vi "run.vi"(8 "error in (no error)":errorcluster, 11 "GenericDisplay in":refnum<class "GenericDisplay.lvclass">) -> (0 "error out":errorcluster, 3 "GenericDisplay out":refnum<class "GenericDisplay.lvclass">)   [LabVIEW 2010, in "GenericDisplay.lvclass"]
uses:
  GenericDisplay.lvclass
panel:
  # "Functionality not available..."
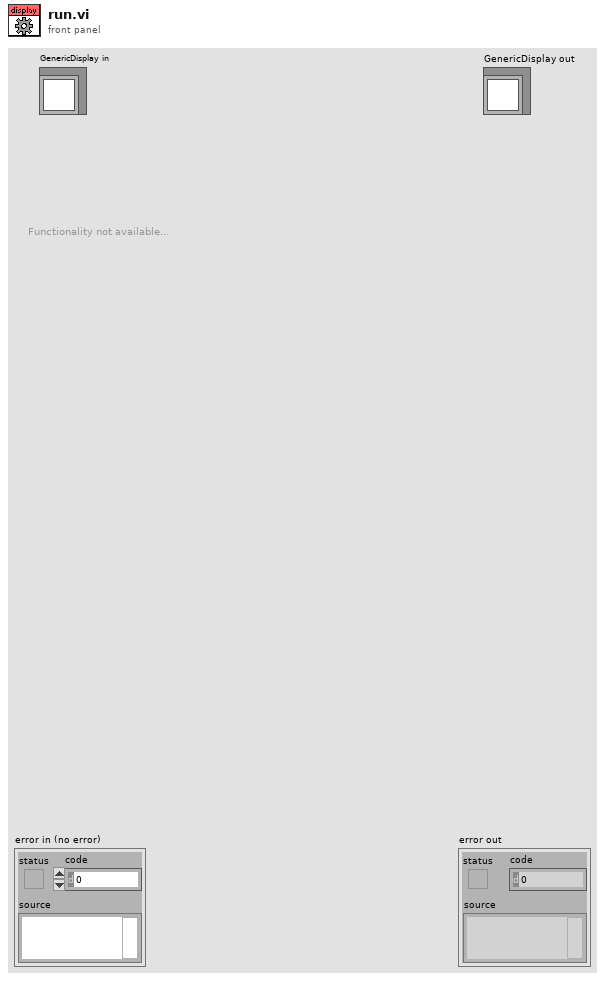
[diagram p1: front panel]
types:
  T1 = typedef "main_trigger_enum.ctl" = enum16{"NULL", "initialise", "terminate", "start", "stop", "change objective", "change experimentController", "change imagingMode", "save notebook", "started saving", "finished saving", "expCtr ready", "expCtr missing", "imgMd ready", "imgMd missing", "scanHd ready", "scanHd missing", "DAQ ready", "DAQ missing", "imgAsm ready", "imgAsm missing", "dataColl ready", "dataColl missing", "display ready", "display missing", "analysr ready", "analysr missing", "instrmnt ready", "instrmnt missing", "stimltr ready", "stimltr missing", "stage ready", "stage missing"}
  T2 = typedef "GenericToplevelComponent.lvclass/common_trigger_enum.ctl" = enum16{"NULL", "initialise", "terminate", "fetch command", "fetch data", "attach observer", "register as observer", "detach observer", "acknowledge", "start", "stop", "sweep started", "sweep finished", "experiment started", "experiment stopped"}
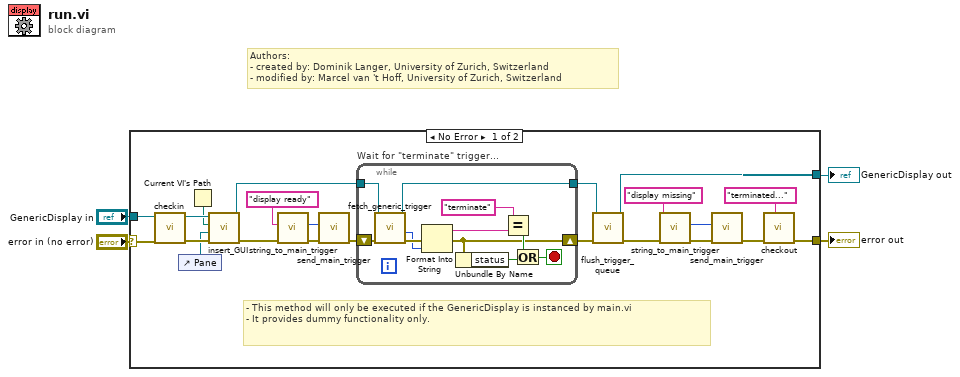
[diagram p0: block diagram]
diagram:
  # "Authors: \n- created by: Dominik Langer, University of Zurich, Switzerland\n- modified by: Marcel van 't Hoff, University of Zurich, Switzerland"
  n1 = case shown="No Error" "error in (no error)" {
    selector: "error in (no error)" -> [w26 w39]
    tunnel: [w23 w39] -> w3
    tunnel: [w14 w38] -> w1
    tunnel: "GenericDisplay in" -> [w25 w38]
    frame No Error {
      # "- This method will only be executed if the GenericDisplay is instanced by main.vi\n- It provides dummy functionality only."
      n2 = call-dynamic "checkin.vi"("error in (no error)"=w26, "GenericDisplay in"=w25) -> ("error out"=w20:errorcluster, "GenericDisplay out"=w21:refnum<class "GenericDisplay.lvclass">)  [unwired: 8 in]
      n3 = control-ref of="Pane"() -> (w18:refnum<vi>)
      n4 = Current VI's Path() -> (path=w19:path)
      n5 = call-dynamic "insert_GUI.vi"("error in (no error)"=w20, "Pane"=w18, "VI path"=w19, "GenericComponent in"=w21) -> ("error out"=w12:errorcluster, "GenericComponent out"=w17:refnum<class "GenericDisplay.lvclass">)  [unwired: 6 in]
      n6 = call "string_to_main_trigger.vi"("error in (no error)"=w12, "trigger string"="display ready") -> ("error out"=w11:errorcluster, "main trigger"=w10:T1)  [unwired: 8 in]
      n7 = call "send_main_trigger.vi"("error in (no error)"=w11, "trigger"=w10) -> ("error out"=w22:errorcluster)  [unwired: 9 in]
      n8 = while "Wait for \"terminate\" trigger..." {
        shift-right: [w30] -> w16
        shift-left: w22 -> [w37]
        tunnel: w17 -> [w36]
        tunnel: [w35] -> w15
        stop <- w32 stop-if-true
        n9 = call-dynamic "fetch_generic_trigger.vi"("error in (no error)"=w37, "GenericToplevelComponent in"=w36) -> ("error out"=w31:errorcluster, "common trigger"=w29:T2, "GenericToplevelComponent out"=w35:refnum<class "GenericDisplay.lvclass">)  [unwired: 3 in, 4 out]
        n10 = Format Into String(error in=w31, w29) -> (resulting string=w28:string, error out=w30:errorcluster)  [unwired: 2 in]
        n11 = Unbundle By Name(w30) -> ("status"=w34:bool)
        n12 = Equal?(x="terminate", y=w28) -> (x = y?=w33:bool)
        n13 = Or(x=w33, y=w34) -> (x .or. y?=w32:bool)
      }
      n14 = call-dynamic "flush_trigger_queue.vi"("error in (no error)"=w16, "GenericToplevelComponent in"=w15) -> ("error out"=w8:errorcluster, "GenericToplevelComponent out"=w14:refnum<class "GenericDisplay.lvclass">)  [unwired: 8 in]
      n15 = call "string_to_main_trigger.vi"("error in (no error)"=w8, "trigger string"="display missing") -> ("error out"=w7:errorcluster, "main trigger"=w5:T1)  [unwired: 8 in]
      n16 = call "send_main_trigger.vi"("error in (no error)"=w7, "trigger"=w5) -> ("error out"=w24:errorcluster)  [unwired: 9 in]
      n17 = call "checkout.vi"("locked by?"="terminated...", "error in (no error)"=w24) -> ("error out"=w23:errorcluster)  [unwired: 8 in, 1 out]
    }
    frame Error {
    }
  }
  "error out" <- w3
  "GenericDisplay out" <- w1
